vi "Create PWM Output Channel.vi"(6 "index":i32, 7 "frequency":T1, 8 "error in":errorcluster, 9 "default value":dbl, 10 "name":string, 11 "PWM output channel in":refnum<class "PWM Output Channel.lvclass">) -> (0 "error out":errorcluster, 3 "PWM output channel out":refnum<class "PWM Output Channel.lvclass">)   [LabVIEW 2017, in "Scan Engine Scripting.lvlib" / "PWM Output Channel.lvclass"]
uses:
  PWM Output Channel.lvclass
  Frequency.ctl
  Channel/Type.ctl
  Channel/Channel.lvclass
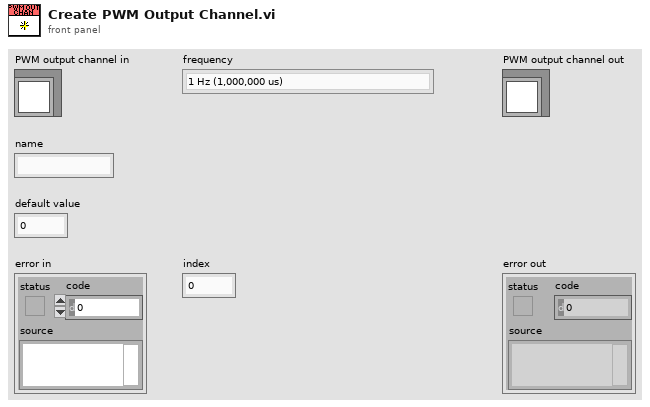
[diagram p1: front panel]
types:
  T1 = typedef "Scan Engine Scripting.lvlib/PWM Output Channel.lvclass/Frequency.ctl" = enum16{"1 Hz (1,000,000 us)", "50 Hz (20,000 us)", "250 Hz (4,000 us)", "500 Hz (2,000 us)", "1 kHz (1,000 us)", "5 kHz (200 us)", "10 kHz (100 us)", "20 kHz (50 us)"}
  T2 = typedef "Scan Engine Scripting.lvlib/Channel.lvclass/Type.ctl" = enum16{"Input", "Output"}
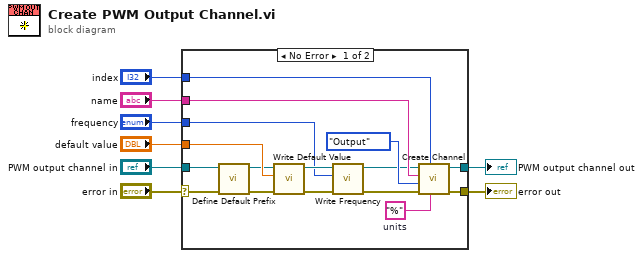
[diagram p0: block diagram]
diagram:
  n1 = case shown="No Error" "error in" {
    selector: "error in" -> [w9 w26]
    tunnel: "default value" -> [w22 _]
    tunnel: "name" -> [w21 _]
    tunnel: "index" -> [w20 _]
    tunnel: [w19 w26] -> w5
    tunnel: [w18 w25] -> w4
    tunnel: "frequency" -> [w13 _]
    tunnel: "PWM output channel in" -> [w12 w25]
    frame No Error {
      w23 = "%"  # units
      n2 = call-dynamic "Define Default Prefix.vi"("error in"=w9, "PWM output channel in"=w12) -> ("error out"=w11:errorcluster, "PWM output channel out"=w10:refnum<class "PWM Output Channel.lvclass">)  [unwired: 8 in]
      n3 = call-dynamic "Write Default Value.vi"("error in"=w11, "default value"=w22, "PWM channel in"=w10) -> ("error out"=w17:errorcluster, "PWM channel out"=w16:refnum<class "PWM Output Channel.lvclass">)  [unwired: 7 in]
      n4 = call-dynamic "Write Frequency.vi"("error in"=w17, "frequency"=w13, "PWM output channel in"=w16) -> ("error out"=w14:errorcluster, "PWM output channel out"=w15:refnum<class "PWM Output Channel.lvclass">)  [unwired: 7 in]
      n5 = call-dynamic "Create Channel.vi"("units"=w23, "index"=w20, "error in"=w14, "type"=Type."Output", "name"=w21, "channel in"=w15) -> ("error out"=w19:errorcluster, "channel out"=w18:refnum<class "PWM Output Channel.lvclass">)  [unwired: 4 in]
    }
    frame Error {
    }
  }
  "error out" <- w5
  "PWM output channel out" <- w4
